vi "Wire ControlReferenceConstants.vi"(8 "error in (no error)":errorcluster, 10 "ControlReferenceConstants":refnum<vi>[](array[refnum]), 11 "NamedBundler":refnum<vi>) -> (0 "error out":errorcluster, 1 "Sorted ControlReferenceConstants":refnum<vi>[](array[refnum]), 2 "Sorted InputTerms[]":refnum<vi>[](array[refnum]))   [LabVIEW 2020, in "Add to Private Data.lvlib"]
uses:
  Add to Private Data.lvlib
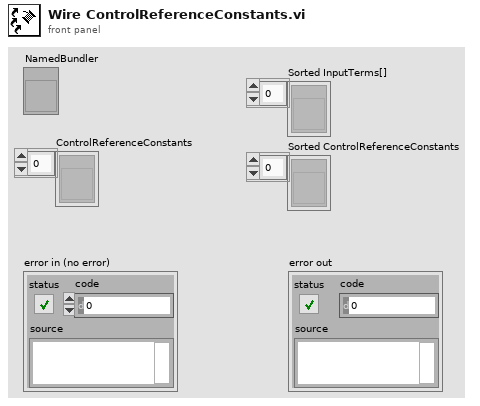
[diagram p1: front panel]
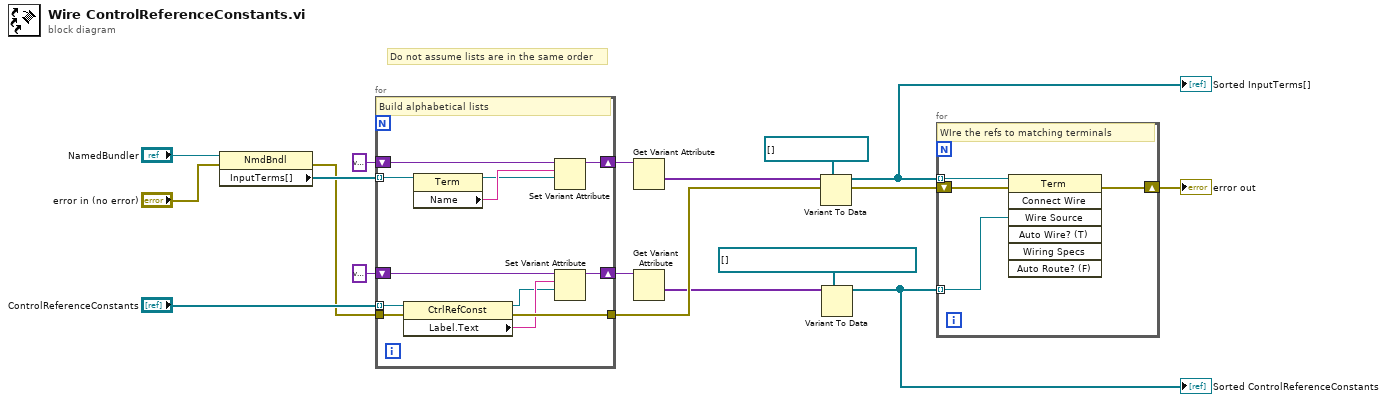
[diagram p0: block diagram]
diagram:
  # "Do not assume lists are in the same order"
  n1 = property class="NmdBndl"(reference="NamedBundler", error in="error in (no error)") -> (error out=w1:errorcluster, "InputTerms[]"=w8:refnum<vi>[])  [unwired: 1 out]
  n2 = for {
    tunnel: "ControlReferenceConstants" -> [w29] mode=indexing
    shift-right: [w28] -> w13
    shift-left: variant -> [w27]
    shift-right: [w25] -> w14
    shift-left: variant -> [w26]
    tunnel: w1 -> [w24]
    tunnel: [w23] -> w10
    tunnel: w8 -> [w21] mode=indexing
    # "Build alphabetical lists"
    n3 = property class="CtrlRefConst"(reference=w29, error in=w24) -> (reference out=w19:refnum<vi>, error out=w23:errorcluster, "Label.Text"=w22:string)
    n4 = property class="Term"(reference=w21) -> (reference out=w18:refnum<vi>, "Name"=w20:string)  [unwired: 1 in, 1 out]
    n5 = Set Variant Attribute(Variant=w26, name=w20, value=w18) -> (Variant out=w25:variant)  [unwired: 1 in, 2 out]
    n6 = Set Variant Attribute(Variant=w27, name=w22, value=w19) -> (Variant out=w28:variant)  [unwired: 1 in, 2 out]
  }
  n7 = Get Variant Attribute(Variant=w14) -> (values=w7:variant[])  [unwired: 3 in, 3 out]
  n8 = Get Variant Attribute(Variant=w13) -> (values=w3:variant[])  [unwired: 3 in, 3 out]
  n9 = Variant To Data(type=refnum<vi>[] [] ("Input Terminals"), Variant=w7) -> (data=w5:refnum<vi>[])  [unwired: 1 in, 1 out]
  "Sorted InputTerms[]" <- w5
  n10 = Variant To Data(type=refnum<vi>[] [] ("ControlReferenceConstants"), Variant=w3) -> (data=w2:refnum<vi>[])  [unwired: 1 in, 1 out]
  "Sorted ControlReferenceConstants" <- w2
  n11 = for {
    tunnel: w5 -> [w31] mode=indexing
    shift-right: [w33] -> w9
    shift-left: w10 -> [w32]
    tunnel: w2 -> [w30] mode=indexing
    # "WIre the refs to matching terminals"
    n12 = invoke class="Term" method="Connect Wire"(reference=w31, error in=w32, "Wire Source"=w30) -> (error out=w33:errorcluster)  [unwired: 4 in, 6 out]
  }
  "error out" <- w9
